vi "Close.vi"(0 "VISA resource name":refnum<visa-resource-name>, 11 "error in (no error)":errorcluster) -> (15 "error out":errorcluster)   [LabVIEW 2012, in "Fluke 5XXX Series Multicalibrators.lvlib"]
doc: "This VI closes the I/O interface with the instrument."
uses:
  Fluke 5XXX Series Multicalibrators.lvlib
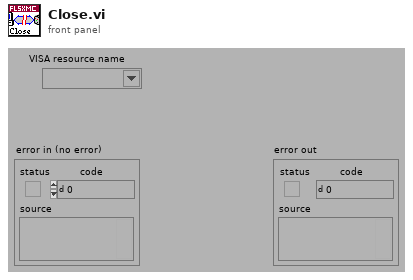
[diagram p1: front panel]
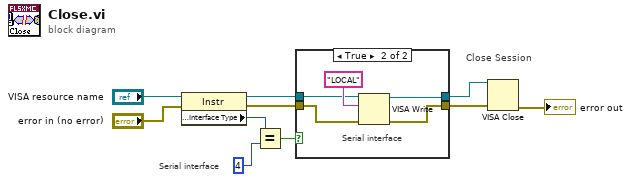
[diagram p0: block diagram]
diagram:
  # "Serial interface"
  # "Close Session"
  n1 = property class="Instr"(reference="VISA resource name", error in="error in (no error)") -> (reference out=w6:refnum<visa-resource-name>, error out=w7:errorcluster, "Interface Information:Interface Type"=w9:u16)
  n2 = Equal?(x=w9, y=u16 4) -> (x = y?=w8:bool)
  n3 = case shown="True" w8 {
    tunnel: w7 -> [w11 w15]
    tunnel: w6 -> [w12 w14]
    tunnel: [w11 w13] -> w4
    tunnel: [w12 w16] -> w3
    frame False {
      # "GPIB interface"
    }
    frame True {
      # "Serial interface"
      n4 = VISA Write(VISA resource name=w14, write buffer="LOCAL" ("ID Query"), error in (no error)=w15) -> (VISA resource name out=w16:refnum<visa-resource-name>, error out=w13:errorcluster)  [unwired: 1 out]
    }
  }
  n5 = VISA Close(VISA resource name=w3, error in (no error)=w4) -> (error out=→"error out":errorcluster)
